vi "Recursive Add Item References to Map.vi"(8 "error in (no error)":errorcluster, 10 "ProjectItem Refnum":refnum<vi>, 11 "Icon Decorator In":refnum<class "Icon Decorator.lvclass">) -> (0 "error out":errorcluster, 3 "Icon Decorator Out":refnum<class "Icon Decorator.lvclass">)   [LabVIEW 2020, in "Icon Decorator.lvlib" / "Icon Decorator.lvclass"]
uses:
  Icon Decorator.lvclass
  Icon Decorator.lvclass/Icon Decorator.ctl
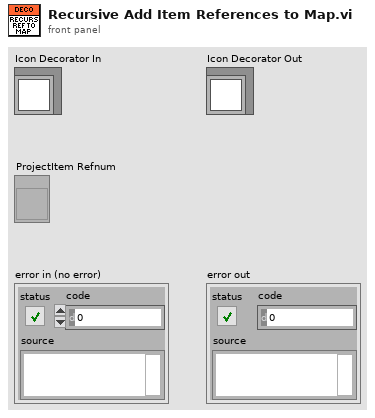
[diagram p1: front panel]
types:
  T1 = typedef "ItemRef.ctl" = u64
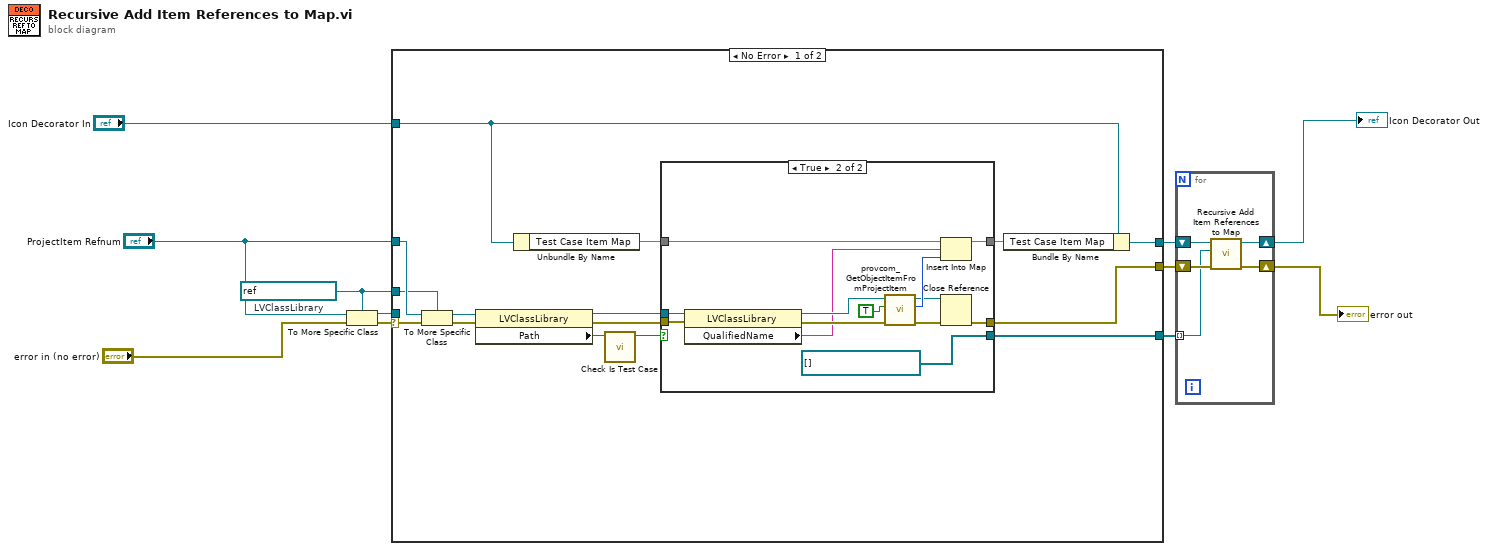
[diagram p0: block diagram]
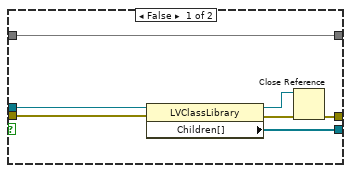
[diagram p2: hidden frame]
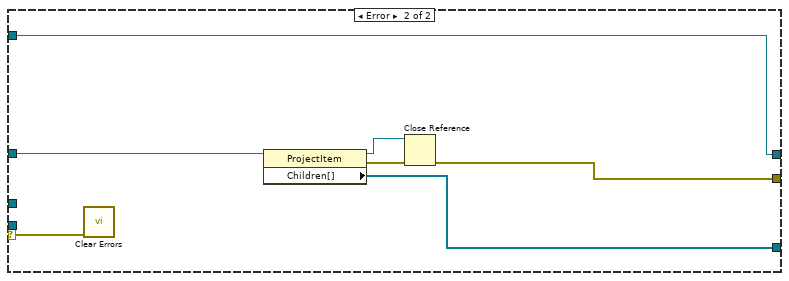
[diagram p3: hidden frame]
diagram:
  w1 = refnum<vi> refnum  # LVClassLibrary
  n1 = To More Specific Class(target class=w1, reference="ProjectItem Refnum", error in="error in (no error)") -> (specific class reference=w3:refnum<vi>, error out=w4:errorcluster)
  n2 = case shown="No Error" w4 {
    selector: w4 -> [w17 w50]
    tunnel: "Icon Decorator In" -> [w26 w47]
    tunnel: [w23 w49] -> w10
    tunnel: [w22 w47] -> w8
    tunnel: [w21 w48] -> w6
    tunnel: w3 -> [_ _]
    tunnel: "ProjectItem Refnum" -> [w13 w51]
    tunnel: w1 -> [w12 _]
    frame No Error {
      n3 = To More Specific Class(target class=w12, reference=w13, error in=w17) -> (specific class reference=w14:refnum<vi>, error out=w15:errorcluster)
      n4 = property class="LVClassLibrary"(reference=w14, error in=w15) -> (reference out=w18:refnum<vi>, error out=w19:errorcluster, "Path"=w20:path)
      n5 = Unbundle By Name(w26) -> ("Test Case Item Map"=w24:map{string, T1})
      n6 = call "Check Is Test Case.vi"("Path"=w20) -> ("Is Test Case?"=w16:bool)  [unwired: 10 in]
      n7 = case shown="True" w16 {
        tunnel: w24 -> [w32 w45]
        tunnel: w18 -> [w29 w44]
        tunnel: w19 -> [w28 w38]
        tunnel: [w33 w40] -> w23
        tunnel: [w32 w39] -> w25
        tunnel: [w27 refnum<vi>[] [] ("Children[]")] -> w21
        frame False {
          n8 = property class="LVClassLibrary"(reference=w29, error in=w28) -> (reference out=w31:refnum<vi>, error out=w30:errorcluster, "Children[]"=w27:refnum<vi>[])
          n9 = Close Reference(reference=w31, error in (no error)=w30) -> (error out=w33:errorcluster)
        }
        frame True {
          n10 = property class="LVClassLibrary"(reference=w44, error in=w38) -> (reference out=w37:refnum<vi>, error out=w36:errorcluster, "QualifiedName"=w35:string)
          n11 = call <resource>:"provcom_GetObjectItemFromProjectItem.vi"("error in (no error)"=w36, "bind? (Y)"=TRUE, "ProjectItem"=w37) -> ("error out"=w41:errorcluster, "ObjectItem"=w43:T1, "dup ProjectItem"=w42:refnum<vi>)  [unwired: 6 in]
          n12 = Insert Into Map(map in=w45, key=w35, value=w43) -> (map out=w39:map{string, T1})  [unwired: 2 out]
          n13 = Close Reference(reference=w42, error in (no error)=w41) -> (error out=w40:errorcluster)
        }
      }
      n14 = Bundle By Name(cluster=w26, "Test Case Item Map"=w25) -> (w22:refnum<class "Icon Decorator.lvclass">)
    }
    frame Error {
      n15 = call <vilib>:"Clear Errors.vi"("error in (no error)"=w50) -> ()  [unwired: 5 in, 2 out]
      n16 = property class="ProjectItem"(reference=w51) -> (reference out=w53:refnum<vi>, error out=w52:errorcluster, "Children[]"=w48:refnum<vi>[])  [unwired: 1 in]
      n17 = Close Reference(reference=w53, error in (no error)=w52) -> (error out=w49:errorcluster)
    }
  }
  n18 = for {
    shift-right: [w57] -> w9
    shift-left: w10 -> [w58]
    shift-right: [w55] -> w7
    shift-left: w8 -> [w56]
    tunnel: w6 -> [w54] mode=indexing
    n19 = call "Recursive Add Item References to Map.vi"("error in (no error)"=w58, "ProjectItem Refnum"=w54, "Icon Decorator In"=w56) -> ("error out"=w57:errorcluster, "Icon Decorator Out"=w55:refnum<class "Icon Decorator.lvclass">)  [unwired: 7 in]
  }
  "Icon Decorator Out" <- w7
  "error out" <- w9
